vi "Solution.vi"() -> ()   [LabVIEW 2020]
panel:
  out "result":i32
  in  "data?":bool
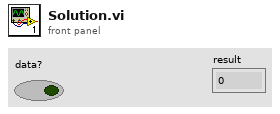
[diagram p1: front panel]
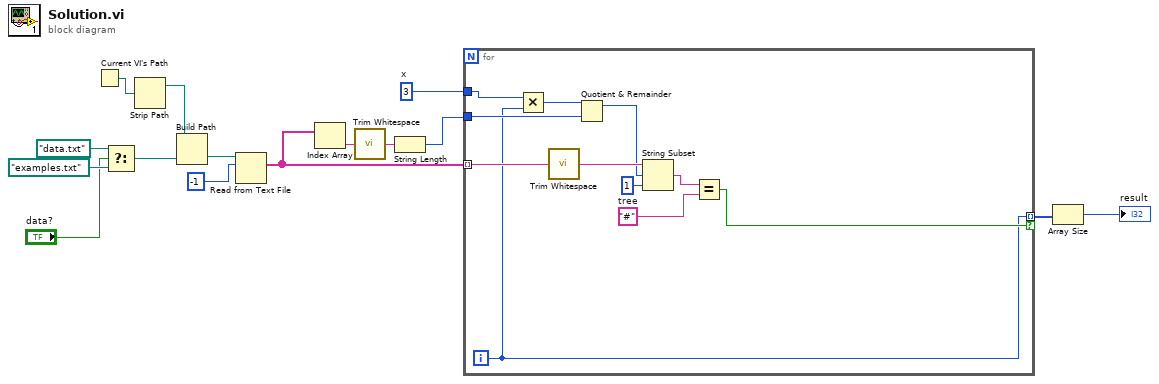
[diagram p0: block diagram]
diagram:
  w2 = 3  # x
  n1 = Current VI's Path() -> (path=w11:path)
  n2 = Select(t=path "data.txt", s="data?", f=path "examples.txt") -> (s? t:f=w12:path)
  n3 = Strip Path(path=w11) -> (stripped path=w10:path)  [unwired: 1 out]
  n4 = Build Path(base path=w10, name or relative path=w12) -> (appended path=w9:path)
  n5 = Read from Text File(file (use dialog)=w9, count=-1) -> (text=w5:string[])  [unwired: 2 in, 3 out]
  n6 = Index Array(array=w5) -> (element=w4:string)  [unwired: 1 in]
  n7 = call <vilib>:"Trim Whitespace.vi"("string"=w4) -> ("trimmed string"=w1:string)  [unwired: 1 in]
  n8 = String Length(string=w1) -> (length=w3:i32)
  n9 = for {
    tunnel: w5 -> [w25] mode=indexing
    tunnel: [w19] -> w8 mode=indexing if=w21
    tunnel: w3 -> [w26]
    tunnel: w2 -> [w18]
    i -> [w19]
    w22 = "#"  # tree
    n10 = Multiply(x=w18, y=w19) -> (x*y=w17:i32)
    n11 = call <vilib>:"Trim Whitespace.vi"("string"=w25) -> ("trimmed string"=w20:string)  [unwired: 1 in]
    n12 = Quotient & Remainder(x=w17, y=w26) -> (x-y*floor(x/y)=w16:i32)  [unwired: 1 out]
    n13 = String Subset(string=w20, offset (0)=w16, length (rest)=1 ("length (rest)")) -> (substring=w23:string)
    n14 = Equal?(x=w23, y=w22) -> (x = y?=w21:bool)
  }
  n15 = Array Size(array=w8) -> (size(s)=→"result":i32)
